vi "Format Plots.vi"(5 "Box Plot Width":dbl=10.0 format="%#_13g", 7 "Line Color":u32(colorbox)=16448250, 8 "error in (no error)":errorcluster, 10 "Number of Plots":i32, 11 "XY Graph":refnum<vi>) -> (0 "error out":errorcluster)   [LabVIEW 2022 SP3, in "Box Plots.lvlib"]
uses:
  Box Plots.lvlib
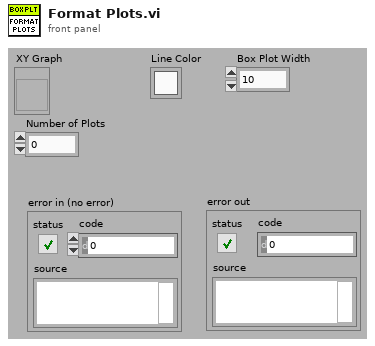
[diagram p1: front panel]
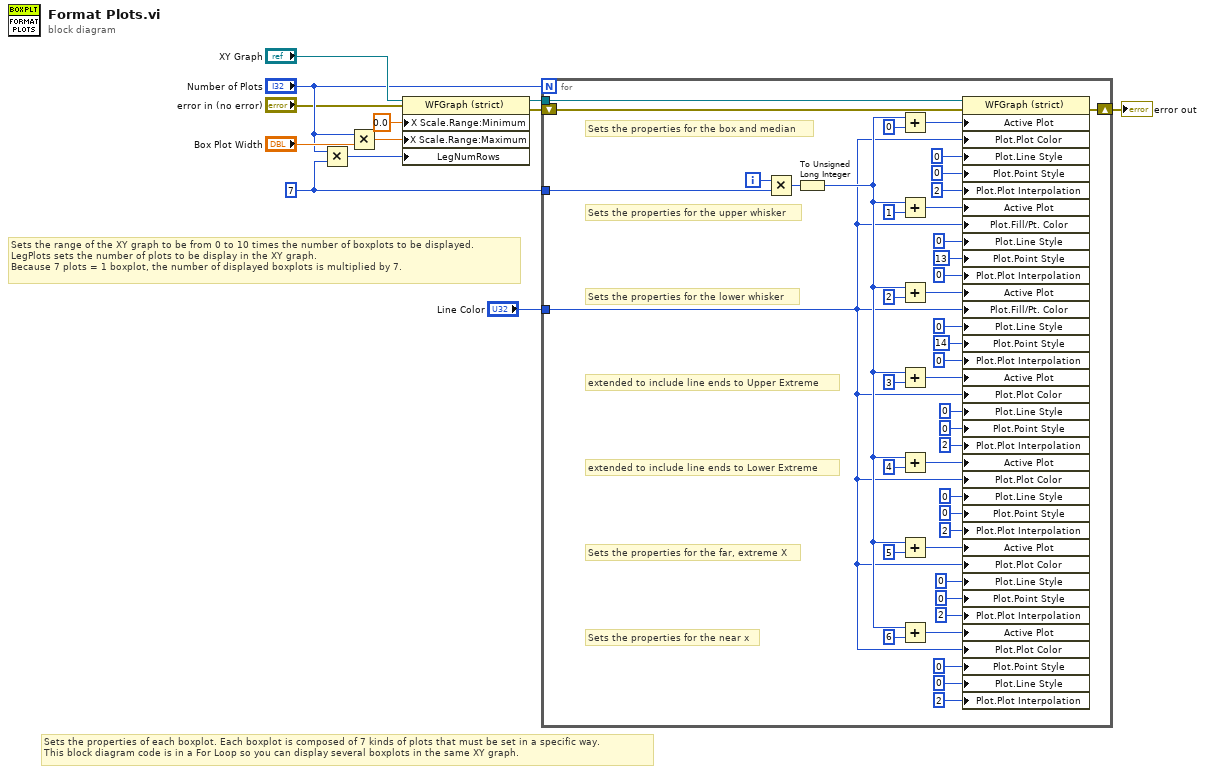
[diagram p0: block diagram]
diagram:
  w4 = 7 ("y")
  # "Sets the range of the XY graph to be from 0 to 10 times the number of boxplots to be displayed.  \nLegPlots sets the number of plots to be display in the XY graph. \nBecause 7 plots = 1 boxplot, the number of displayed boxplots is multiplied by 7."
  # "Sets the properties of each boxplot. Each boxplot is composed of 7 kinds of plots that must be set in a specific way. \nThis block diagram code is in a For Loop so you can display several boxplots in the same XY graph."
  n1 = Multiply(x="Number of Plots", y=w4) -> (x*y=w12:i32)
  n2 = Multiply(x="Number of Plots", y="Box Plot Width") -> (x*y=w9:dbl)
  n3 = property on="Property Node" class="WFGraph (strict)"(reference="XY Graph", error in="error in (no error)", "X Scale.Range:Minimum"=0.0 ("Legend:Plots Shown"), "X Scale.Range:Maximum"=w9, "LegNumRows"=w12) -> (reference out=w8:refnum<vi>, error out=w5:errorcluster)
  n4 = for {
    N: "Number of Plots" -> [_]
    tunnel: w8 -> [w55]
    shift-right: [w30] -> w3
    shift-left: w5 -> [w48]
    tunnel: w4 -> [w14]
    tunnel: "Line Color" -> [w13]
    i -> [w51]
    # "Sets the properties for the box and median"
    # "Sets the properties for the near x"
    # "Sets the properties for the far, extreme X"
    # "extended to include line ends to Upper Extreme"
    # "extended to include line ends to Lower Extreme"
    # "Sets the properties for the lower whisker"
    # "Sets the properties for the upper whisker"
    n5 = Multiply(x=w51, y=w14) -> (x*y=w24:i32)
    n6 = To Unsigned Long Integer(number=w24) -> (unsigned 32bit integer=w15:u32)
    n7 = Add(x=w15, y=u32 0) -> (x+y=w53:u32)
    n8 = Add(x=w15, y=u32 1) -> (x+y=w46:u32)
    n9 = Add(x=w15, y=u32 2) -> (x+y=w40:u32)
    n10 = Add(x=w15, y=u32 3) -> (x+y=w36:u32)
    n11 = Add(x=w15, y=u32 4) -> (x+y=w31:u32)
    n12 = Add(x=w15, y=u32 5) -> (x+y=w28:u32)
    n13 = Add(x=w15, y=u32 6) -> (x+y=w23:u32)
    n14 = property on="Property Node" class="WFGraph (strict)"(reference=w55, error in=w48, "Active Plot"=w53, "Plot.Plot Color"=w13, "Plot.Line Style"=u8 0, "Plot.Point Style"=u8 0, "Plot.Plot Interpolation"=u8 2, "Active Plot"=w46, "Plot.Fill/Pt. Color"=w13, "Plot.Line Style"=u8 0 ("Plot.Line Style 2"), "Plot.Point Style"=u8 13 ("Plot.Point Style 2"), "Plot.Plot Interpolation"=u8 0 ("Active Cursor"), "Active Plot"=w40, "Plot.Fill/Pt. Color"=w13, "Plot.Line Style"=u8 0 ("Plot.Line Style 3"), "Plot.Point Style"=u8 14 ("Plot.Point Style 3"), "Plot.Plot Interpolation"=u8 0, "Active Plot"=w36, "Plot.Plot Color"=w13, "Plot.Line Style"=u8 0 ("Plot.Line Style 4"), "Plot.Point Style"=u8 0 ("Plot.Point Style 4"), "Plot.Plot Interpolation"=u8 2, "Active Plot"=w31, "Plot.Plot Color"=w13, "Plot.Line Style"=u8 0 ("Plot.Line Style 5"), "Plot.Point Style"=u8 0 ("Plot.Point Style 5"), "Plot.Plot Interpolation"=u8 2, "Active Plot"=w28, "Plot.Plot Color"=w13, "Plot.Line Style"=u8 0 ("Plot.Line Style 5"), "Plot.Point Style"=u8 0 ("Plot.Point Style 5"), "Plot.Plot Interpolation"=u8 2, "Active Plot"=w23, "Plot.Plot Color"=w13, "Plot.Point Style"=u8 0 ("Plot.Point Style 5"), "Plot.Line Style"=u8 0 ("Plot.Line Style 5"), "Plot.Plot Interpolation"=u8 2) -> (error out=w30:errorcluster)  [unwired: 1 out]
  }
  "error out" <- w3
